vi "ParseTest.vi"(11 "Responce":string="\u000201AMI,OK,TEMP-2000  V00-R0024\r\n") -> (1 "Payload":string, 2 "Command":string, 3 "Address":u8, 5 "OK":bool, 7 "Checksum OK":bool)   [LabVIEW 2015]
uses:
  <instrlib>/Samwontech TEMP2xxx/Samwontech TEMP2xxx.lvlib
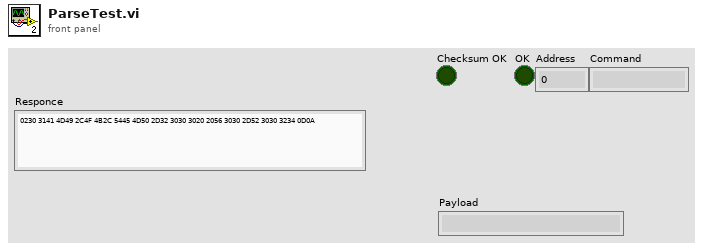
[diagram p1: front panel]
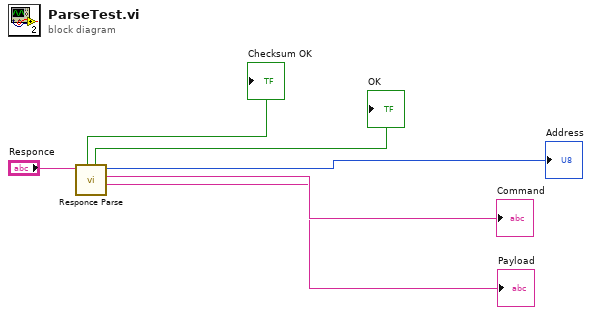
[diagram p0: block diagram]
diagram:
  n1 = call <instrlib>:"Responce Parse.vi"("Responce"="Responce") -> ("Payload"=→"Payload":string, "Command"=→"Command":string, "Address"=→"Address":u8, "OK"=→"OK":bool, "Checksum OK"=→"Checksum OK":bool)  [unwired: 4 in, 2 out]
